vi "Serialize To Inputs.vi"(0 "Input 6":variant, 4 "Input 5":variant, 6 "Input 4":variant, 8 "Input 3":variant, 9 "Input 2":variant, 10 "Input 1":variant, 11 "jettl in":refnum<class "jettl.lvclass">) -> (3 "jettl out":refnum<class "jettl.lvclass">)   [LabVIEW 2021, in "jettl.lvlib" / "jettl.lvclass"]
uses:
  jettl.lvclass
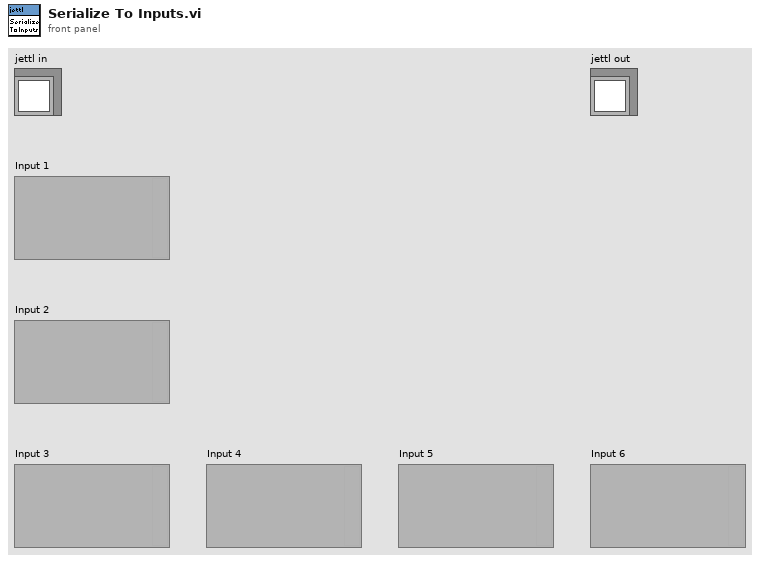
[diagram p1: front panel]
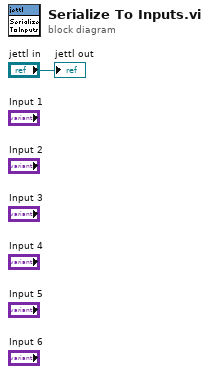
[diagram p0: block diagram]
diagram:
  "jettl out" <- "jettl in"
